vi "Build Test Node Directory Path.vi"(11 "Project Path":path) -> (3 "Test Node Directory Path":path)   [LabVIEW 2013, in "File IO.lvlib"]
uses:
  File IO.lvlib
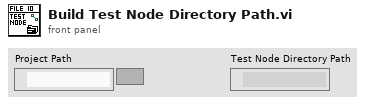
[diagram p1: front panel]
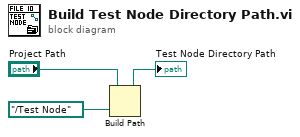
[diagram p0: block diagram]
diagram:
  n1 = Build Path(base path="Project Path", name or relative path=path "../Test Node") -> (appended path=→"Test Node Directory Path":path)
